vi "Main.vi"() -> ()   [LabVIEW 2021]
uses:
  Type defs/timer Indicator.ctl
  Type defs/Boolean References.ctl
  Type defs/numeric references.ctl
  Type defs/States.ctl
  Type defs/Game Config.ctl
  Type defs/Logs Array.ctl
  <vilib>/Utility/file.llb/Write Delimited Spreadsheet (string).vi
panel:
  in  "increment":bool
  out "Time":string
  in  "Game Config":T1={"Foul Limits"=5.0, "Timeouts Allowed"=5.0, "Game time"=5.0} {"Game time" format="%#_g Min"}
  out "Game Status":enum16{"Paused", "Resumed"}(ring)
  out "Current State":T2
  out "File Status":errorcluster
  out "No. of events Logged":i32
  out "Logging path chosen":path
  out "Logs":string[](array[string])
  in  "Log file path":path
  out "Scores History":dbl[][](graph)
  out "Numeric References":T3
  out "Boolean Refernces":T4
  out "Quarter":dbl
  out "no_timeouts_B":bool
  out "no_timeouts_A":bool
  out "Timeouts_B":dbl
  out "Timeouts_A":dbl
  out "Fouls_Limit B":bool
  out "Fouls_Limit A":bool
  out "Fouls_B":dbl
  out "Fouls_A":dbl
  out "quarter_score_B":dbl[](array[numeric])
  out "quarter_score_A":dbl[](array[numeric])
  out "Score_B":dbl
  out "Score_A":dbl
  in  "Save Logs":bool
  in  "Reset":bool
  in  "Advance Quarter":bool
  in  "Start/Pause":bool
  in  "B_timeout":bool
  in  "B_Foul":bool
  in  "B_3pt":bool
  in  "B_2pt":bool
  in  "B_1pt":bool
  in  "A_timeout":bool
  in  "A_Foul":bool
  in  "A_3pt":bool
  in  "A_2pt":bool
  in  "A_1pt":bool
  out "Timer":T5
  in  "Stop":bool
  # "Game Status"
  # "TEAM B"
  # "TEAM A"
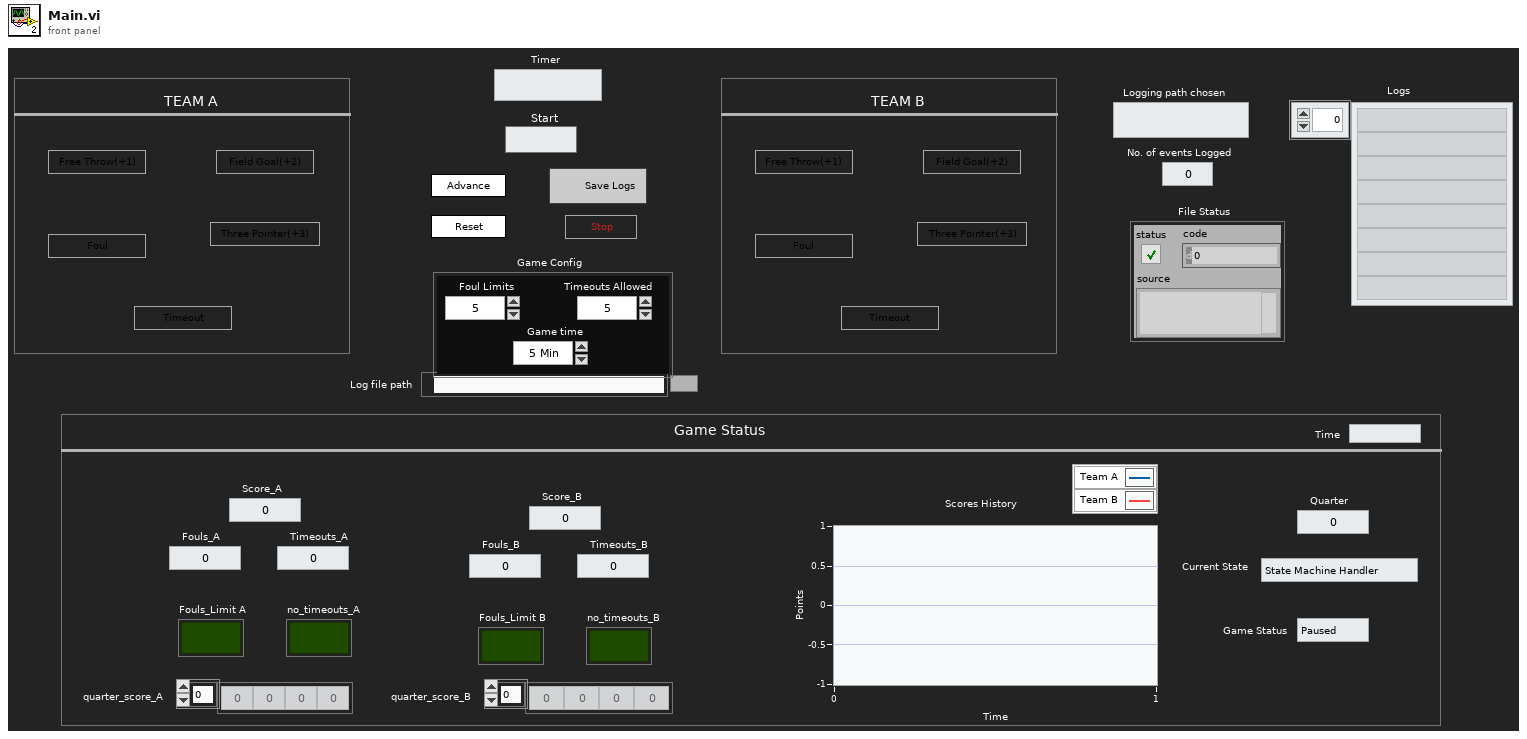
[diagram p1: front panel]
types:
  T1 = typedef "Game Config.ctl" = cluster{"Foul Limits":dbl, "Timeouts Allowed":dbl, "Game time":dbl}
  T2 = typedef "States.ctl" = enum16{"State Machine Handler", "A_1pt", "B_1pt", "A_2pt", "B_2pt", "A_3pt", "B_3pt", "A_Foul", "B_Foul", "A_timeout", "B_timeout", "Next Quarter", "Save Logs", "Reset", "Start/Pause", "Stop"}
  T3 = typedef "numeric references.ctl" = refnum<vi>[]
  T4 = typedef "Boolean References.ctl" = refnum<vi>[]
  T5 = typedef "timer Indicator.ctl" = string
  T6 = typedef "Logs Array.ctl" = string[]
  T7 = enum8{"Enabled", "Disabled", "Disabled and Grayed Out"}
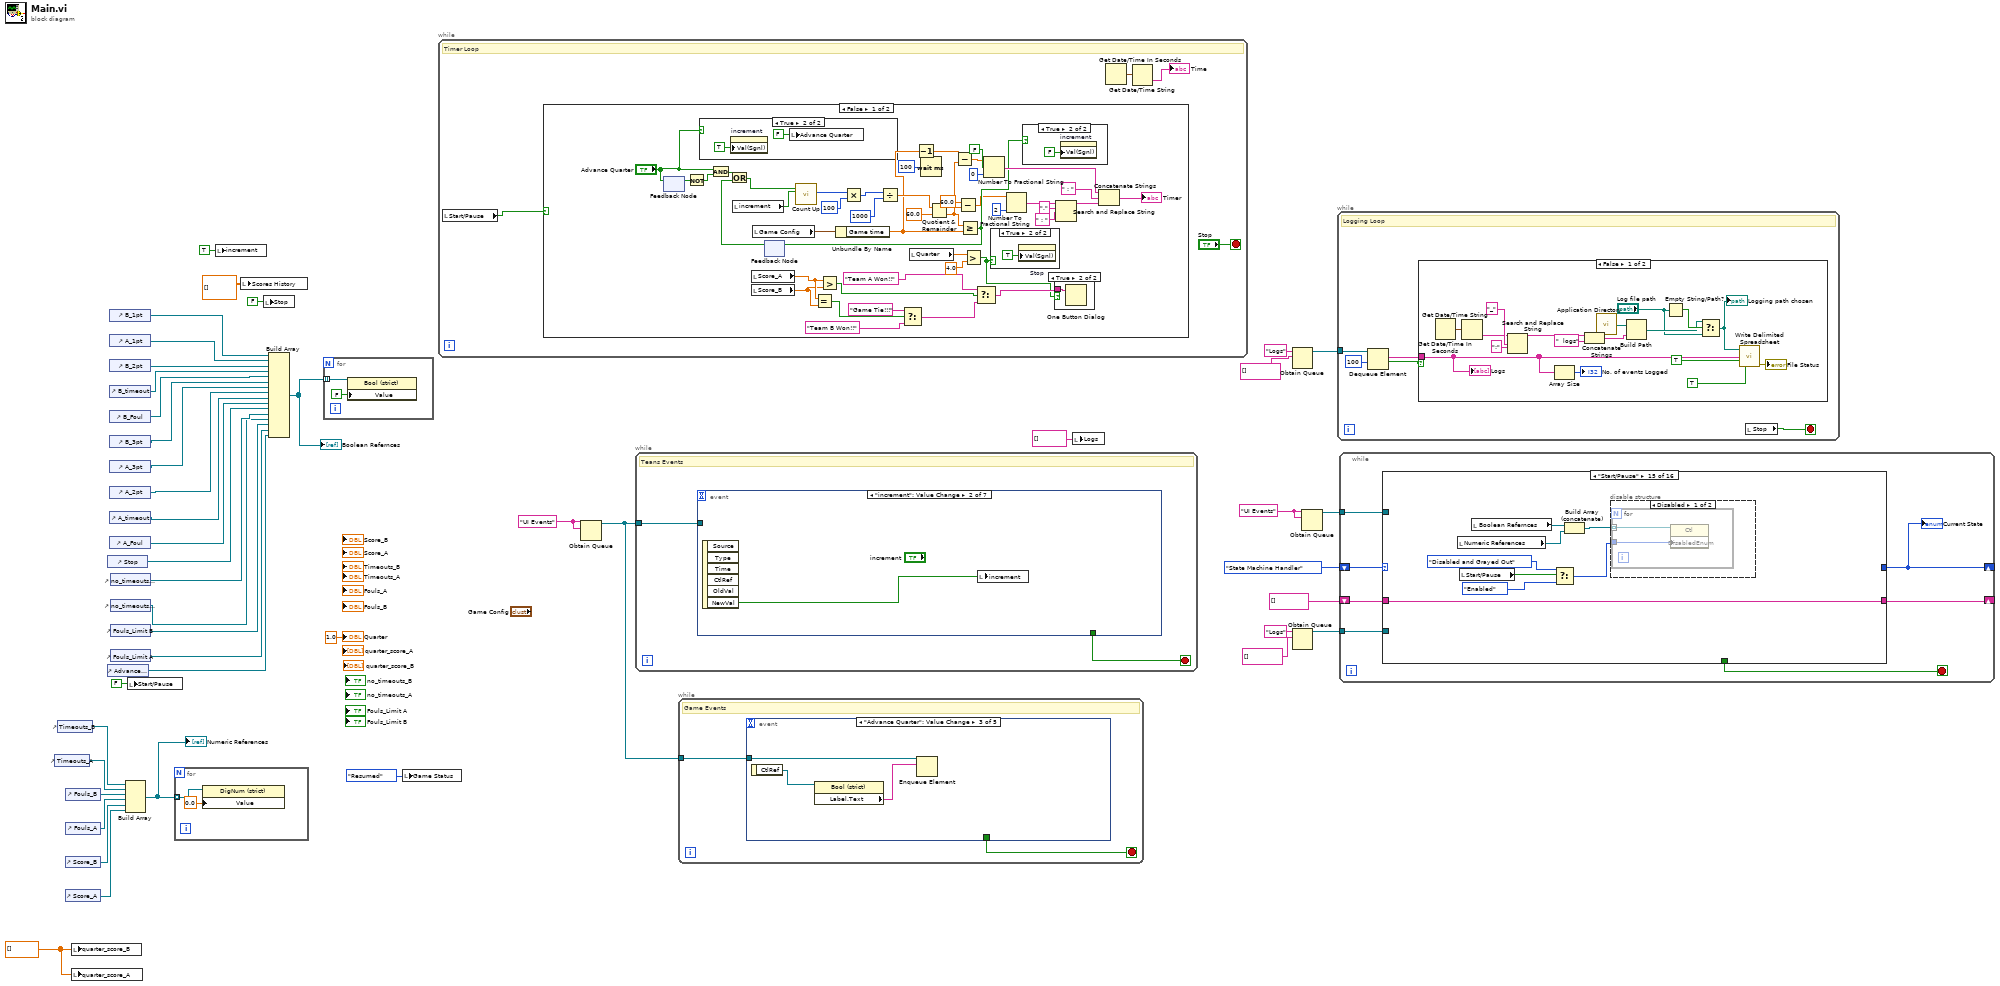
[diagram p0: block diagram]
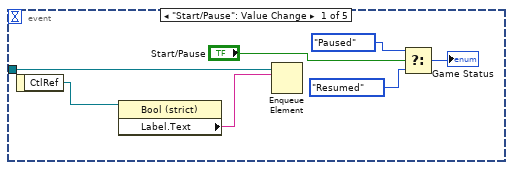
[diagram p2: hidden frame]
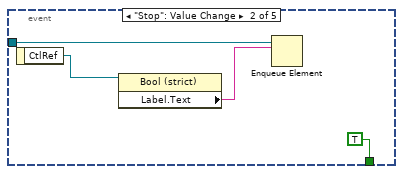
[diagram p3: hidden frame]
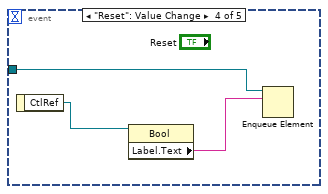
[diagram p4: hidden frame]
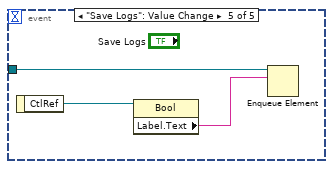
[diagram p5: hidden frame]
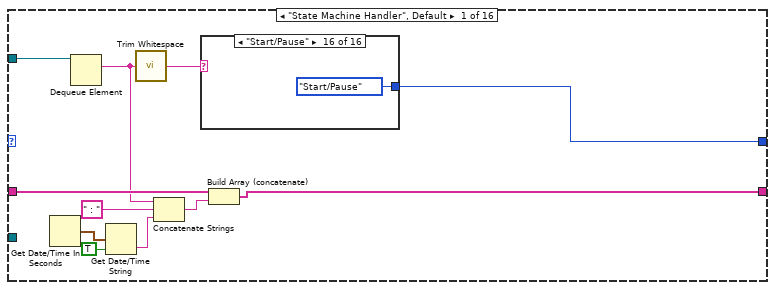
[diagram p6: hidden frame]
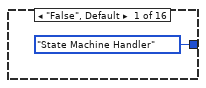
[diagram p7: hidden frame]
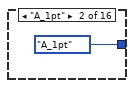
[diagram p8: hidden frame]
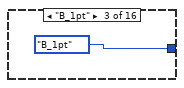
[diagram p9: hidden frame]
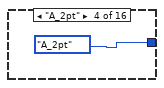
[diagram p10: hidden frame]
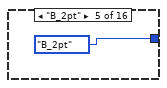
[diagram p11: hidden frame]
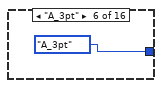
[diagram p12: hidden frame]
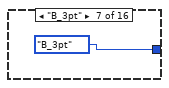
[diagram p13: hidden frame]
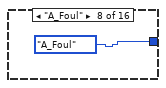
[diagram p14: hidden frame]
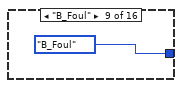
[diagram p15: hidden frame]
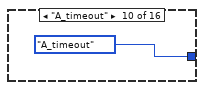
[diagram p16: hidden frame]
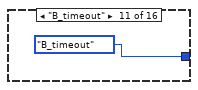
[diagram p17: hidden frame]
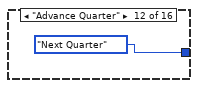
[diagram p18: hidden frame]
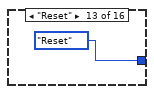
[diagram p19: hidden frame]
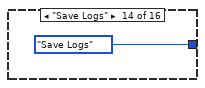
[diagram p20: hidden frame]
diagram:
  w17 = dbl[] [] ("quarter_score_B")
  w32 = "UI Events" ("Label.Text")
  w33 = "UI Events" ("Label.Text")
  n1 = control-ref of="Timeouts_A"() -> (w23:refnum<vi>)
  n2 = control-ref of="Timeouts_B"() -> (w24:refnum<vi>)
  n3 = control-ref of="Fouls_B"() -> (w22:refnum<vi>)
  n4 = control-ref of="Fouls_A"() -> (w21:refnum<vi>)
  n5 = control-ref of="Score_B"() -> (w20:refnum<vi>)
  n6 = control-ref of="Score_A"() -> (w19:refnum<vi>)
  n7 = local write "quarter_score_B"(w17) -> ()
  n8 = local write "quarter_score_A"(w17) -> ()
  n9 = control-ref of="Stop"() -> (w29:refnum<vi>)
  n10 = control-ref of="Advance Quarter"() -> (w3:refnum<vi>)
  n11 = control-ref of="B_1pt"() -> (w44:refnum<vi>)
  n12 = control-ref of="A_1pt"() -> (w43:refnum<vi>)
  n13 = control-ref of="B_2pt"() -> (w42:refnum<vi>)
  n14 = control-ref of="B_timeout"() -> (w41:refnum<vi>)
  n15 = control-ref of="B_Foul"() -> (w40:refnum<vi>)
  n16 = control-ref of="B_3pt"() -> (w39:refnum<vi>)
  n17 = control-ref of="A_3pt"() -> (w38:refnum<vi>)
  n18 = control-ref of="A_2pt"() -> (w37:refnum<vi>)
  n19 = control-ref of="A_timeout"() -> (w36:refnum<vi>)
  n20 = control-ref of="A_Foul"() -> (w35:refnum<vi>)
  n21 = control-ref of="no_timeouts_B"() -> (w28:refnum<vi>)
  n22 = control-ref of="no_timeouts_A"() -> (w27:refnum<vi>)
  n23 = control-ref of="Fouls_Limit B"() -> (w26:refnum<vi>)
  n24 = control-ref of="Fouls_Limit A"() -> (w25:refnum<vi>)
  n25 = Build Array(w24, w23, w22, w21, w20, w19) -> (w18:refnum<vi>[])
  "Numeric References" <- w18
  n26 = local write "Start/Pause"(FALSE ("Start/Pause")) -> ()
  n27 = for {
    tunnel: w18 -> [w46] mode=indexing
    n28 = property class="DigNum (strict)"(reference=w46, "Value"=0.0) -> ()  [unwired: 1 in, 2 out]
  }
  n29 = local write "increment"(TRUE ("increment")) -> ()
  n30 = local write "Scores History"(dbl[][] [] ("Scores History")) -> ()
  n31 = local write "Stop"(FALSE ("Stop")) -> ()
  n32 = Build Array(w44, w43, w42, w41, w40, w39, w38, w37, w36, w35, w29, w28, w27, w26, w25, w3) -> (w34:refnum<vi>[])
  "Boolean Refernces" <- w34
  n33 = for {
    tunnel: w34 -> [w48] mode=indexing
    n34 = property class="Bool (strict)"(reference=w48, "Value"=FALSE) -> ()  [unwired: 1 in, 2 out]
  }
  n35 = local write "Game Status"(enum16{"Paused", "Resumed"}."Resumed" ("Game Status")) -> ()
  n36 = while {
    stop <- "Stop" stop-if-true
    # "Timer Loop"
    n37 = local read "Start/Pause"() -> (w49:bool)
    n38 = case shown="False" w49 {
      frame False {
        n39 = feedback #1() -> (w65:bool)  [unwired: 1 in]
        n40 = feedback-in #1("Advance Quarter") -> ()
        n41 = Not(x=w65) -> (.not. x?=w64:bool)
        n42 = case shown="True" "Advance Quarter" {
          frame False {
          }
          frame True {
            n43 = property on="increment" class="Bool (strict)"("Val(Sgnl)"=TRUE ("Value (Signaling)")) -> ()  [unwired: 2 in, 2 out]
            n44 = local write "Advance Quarter"(FALSE ("Advance Quarter")) -> ()
          }
        }
        n45 = And(x="Advance Quarter", y=w64) -> (x .and. y?=w66:bool)
        n46 = local read "increment"() -> (w60:bool)
        n47 = local read "Score_A"() -> (w80:dbl)
        n48 = local read "Score_B"() -> (w79:dbl)
        n49 = local read "Game Config"() -> (w68:T1)
        n50 = feedback #2() -> (w62:bool)  [unwired: 1 in]
        n51 = Or(x=w66, y=w62) -> (x .or. y?=w67:bool)
        n52 = call "Count Up.vi"("Reset"=w67, "Increment"=w60) -> ("Count"=w74:i32)  [unwired: 9 in]
        n53 = Equal?(x=w80, y=w79) -> (x = y?=w78:bool)
        n54 = Greater?(x=w80, y=w79) -> (0:w81:bool)
        n55 = Unbundle By Name(w68) -> ("Game time"=w59:dbl)
        n56 = Multiply(x=w74, y=100) -> (x*y=w73:i32)
        n57 = Divide(x=w73, y=u32 1000) -> (x/y=w90:dbl)
        n58 = Select(t="Game Tie!!!", s=w78, f="Team B Won!!" ("replace string (\"\")")) -> (s? t:f=w75:string)
        n59 = local read "Quarter"() -> (w71:dbl)
        n60 = Decrement(x=w59) -> (x-1=w53:dbl)
        n61 = Wait (ms)(milliseconds to wait=u32 100) -> ()  [unwired: 1 out]
        n62 = Quotient & Remainder(x=w90, y=60.0) -> (x-y*floor(x/y)=w56:dbl, floor(x/y)=w58:dbl)
        n63 = Subtract(x=w53, y=w58) -> (x-y=w57:dbl)
        n64 = Subtract(x=60.0, y=w56) -> (x-y=w54:dbl)
        n65 = Greater Or Equal?(x=w58, y=w59) -> (x >= y?=w61:bool)
        n66 = feedback-in #2(w61) -> ()
        n67 = Greater?(x=w71, y=4.0) -> (0:w69:bool)
        n68 = Select(t="Team A Won!!" ("replace string (\"\")"), s=w81, f=w75) -> (s? t:f=w82:string)
        n69 = Number To Fractional String(use system decimal point (T)=FALSE, number=w57, precision (6)=i16 0) -> (F-format string=w85:string)  [unwired: 1 in]
        n70 = case shown="True" w69 {
          frame False {
          }
          frame True {
            n71 = property on="Stop" class="Bool (strict)"("Val(Sgnl)"=TRUE ("Value (Signaling)")) -> ()  [unwired: 2 in, 2 out]
          }
        }
        n72 = Number To Fractional String(number=w54, precision (6)=i16 2) -> (F-format string=w94:string)  [unwired: 2 in]
        n73 = case shown="True" w61 {
          frame False {
          }
          frame True {
            n74 = property on="increment" class="Bool (strict)"("Val(Sgnl)"=FALSE ("Value (Signaling)")) -> ()  [unwired: 2 in, 2 out]
          }
        }
        n75 = case shown="True" w69 {
          tunnel: w82 -> [_ w101]
          frame False {
          }
          frame True {
            n76 = One Button Dialog(message=w101) -> ()  [unwired: 1 in, 1 out]
          }
        }
        n77 = Search and Replace String(input string=w94, search string=".", replace string=" : " ("replace string (\"\")")) -> (result string=w91:string)  [unwired: 5 in, 3 out]
        n78 = Concatenate Strings(w85, " : " ("replace string (\"\")"), w91) -> (→"Timer":string)
      }
      frame True {
      }
    }
    n79 = Get Date/Time In Seconds() -> (seconds since 1Jan1904=w51:timestamp)
    n80 = Get Date/Time String(seconds (now)=w51) -> (time string=→"Time":string)  [unwired: 2 in, 1 out]
  }
  n81 = Obtain Queue(name (unnamed)=w33, element data type=w33) -> (queue out=w10:refnum<queue>)  [unwired: 3 in, 2 out]
  n82 = while {
    tunnel: w10 -> [w104]
    stop <- w103 stop-if-true
    # "Teans Events"
    n83 = event shown="[1] \"increment\": Value Change" {
      selector: _ -> [_ _ _ _ _ _ _]
      dyn-events: _ -> [_ _ _ _ _ _ _]
      timeout: _ -> [_ _ _ _ _ _ _]
      tunnel: w104 -> [w107 _ w113 w115 w118 w122 w125]
      tunnel: [w105 _ _ _ _ _ _] -> w103
      event "Stop": Value Change {
        n84 = event-data() -> ("CtlRef"=w106:refnum<vi>)  [unwired: 1 in, 2 out]
        n85 = disable-structure shown="Enabled" {
          disable-tunnel: w107 -> [w109 _]
          disable-tunnel: w106 -> [w108 _]
          frame Enabled {
            n86 = property class="Bool (strict)"(reference=w108) -> ("Label.Text"=w110:string)  [unwired: 1 in, 2 out]
            n87 = Enqueue Element(queue=w109, element=w110) -> ()  [unwired: 2 in, 3 out]
          }
          frame Disabled {
          }
        }
        n88 = local read "Stop"() -> (w105:bool)
      }
      event "increment": Value Change {
        n89 = event-data() -> ("NewVal"=w111:bool)  [unwired: 1 in, 5 out]
        n90 = local write "increment"(w111) -> ()
      }
      event "A_1pt", "B_1pt": Value Change {
        n91 = event-data() -> ("CtlRef"=w114:refnum<vi>)  [unwired: 1 in]
        n92 = property class="Bool (strict)"(reference=w114) -> ("Label.Text"=w112:string)  [unwired: 1 in, 2 out]
        n93 = Enqueue Element(queue=w113, element=w112) -> ()  [unwired: 2 in, 3 out]
      }
      event "A_2pt", "B_2pt": Value Change {
        n94 = event-data() -> ("CtlRef"=w116:refnum<vi>)  [unwired: 1 in, 2 out]
        n95 = property class="Bool (strict)"(reference=w116) -> ("Label.Text"=w117:string)  [unwired: 1 in, 2 out]
        n96 = Enqueue Element(queue=w115, element=w117) -> ()  [unwired: 2 in, 3 out]
      }
      event "A_3pt", "B_3pt": Value Change {
        n97 = event-data() -> ("CtlRef"=w119:refnum<vi>)  [unwired: 1 in, 2 out]
        n98 = property class="Bool (strict)"(reference=w119) -> ("Label.Text"=w120:string)  [unwired: 1 in, 2 out]
        n99 = Enqueue Element(queue=w118, element=w120) -> ()  [unwired: 2 in, 3 out]
      }
      event "A_Foul", "B_Foul": Value Change {
        n100 = event-data() -> ("CtlRef"=w121:refnum<vi>)  [unwired: 1 in, 2 out]
        n101 = property class="Bool (strict)"(reference=w121) -> ("Label.Text"=w123:string)  [unwired: 1 in, 2 out]
        n102 = Enqueue Element(queue=w122, element=w123) -> ()  [unwired: 2 in, 3 out]
      }
      event "A_timeout", "B_timeout": Value Change {
        n103 = event-data() -> ("CtlRef"=w124:refnum<vi>)  [unwired: 1 in, 2 out]
        n104 = property class="Bool (strict)"(reference=w124) -> ("Label.Text"=w126:string)  [unwired: 1 in, 2 out]
        n105 = Enqueue Element(queue=w125, element=w126) -> ()  [unwired: 2 in, 3 out]
      }
    }
  }
  n106 = while {
    tunnel: w10 -> [w128]
    stop <- w127 stop-if-true
    # "Game Events"
    n107 = event shown="[2] \"Advance Quarter\": Value Change" {
      selector: _ -> [_ _ _ _ _]
      dyn-events: _ -> [_ _ _ _ _]
      timeout: _ -> [_ _ _ _ _]
      tunnel: w128 -> [w133 w137 w140 w144 w147]
      tunnel: [_ TRUE _ _ _] -> w127
      event "Start/Pause": Value Change {
        n108 = event-data() -> ("CtlRef"=w134:refnum<vi>)  [unwired: 1 in]
        n109 = property class="Bool (strict)"(reference=w134) -> ("Label.Text"=w135:string)  [unwired: 1 in, 2 out]
        n110 = Enqueue Element(queue=w133, element=w135) -> ()  [unwired: 2 in, 3 out]
        n111 = Select(t=enum16{"Paused", "Resumed"}."Paused", s="Start/Pause", f=enum16{"Paused", "Resumed"}."Resumed") -> (s? t:f=→"Game Status":enum16{"Paused", "Resumed"})
      }
      event "Stop": Value Change {
        n112 = event-data() -> ("CtlRef"=w138:refnum<vi>)  [unwired: 1 in]
        n113 = property class="Bool (strict)"(reference=w138) -> ("Label.Text"=w139:string)  [unwired: 1 in, 2 out]
        n114 = Enqueue Element(queue=w137, element=w139) -> ()  [unwired: 2 in, 3 out]
      }
      event "Advance Quarter": Value Change {
        n115 = event-data() -> ("CtlRef"=w141:refnum<vi>)  [unwired: 1 in]
        n116 = property class="Bool (strict)"(reference=w141) -> ("Label.Text"=w142:string)  [unwired: 1 in, 2 out]
        n117 = Enqueue Element(queue=w140, element=w142) -> ()  [unwired: 2 in, 3 out]
      }
      event "Reset": Value Change {
        n118 = event-data() -> ("CtlRef"=w143:refnum<vi>)  [unwired: 1 in]
        n119 = property class="Bool"(reference=w143) -> ("Label.Text"=w145:string)  [unwired: 1 in, 2 out]
        n120 = Enqueue Element(queue=w144, element=w145) -> ()  [unwired: 2 in, 3 out]
      }
      event "Save Logs": Value Change {
        n121 = event-data() -> ("CtlRef"=w146:refnum<vi>)  [unwired: 1 in]
        n122 = property class="Bool"(reference=w146) -> ("Label.Text"=w148:string)  [unwired: 1 in, 2 out]
        n123 = Enqueue Element(queue=w147, element=w148) -> ()  [unwired: 2 in, 3 out]
      }
    }
  }
  n124 = local write "Logs"(string[] [] ("Logs")) -> ()
  n125 = Obtain Queue(name (unnamed)="Logs", element data type=T6 []) -> (queue out=w11:refnum<queue>)  [unwired: 3 in, 2 out]
  n126 = Obtain Queue(name (unnamed)="Logs", element data type=T6 []) -> (queue out=w13:refnum<queue>)  [unwired: 3 in, 2 out]
  n127 = Obtain Queue(name (unnamed)=w32, element data type=w32) -> (queue out=w31:refnum<queue>)  [unwired: 3 in, 2 out]
  n128 = while {
    tunnel: w11 -> [w152]
    stop <- w153 stop-if-true
    # "Logging Loop"
    n129 = Dequeue Element(queue=w152, timeout in ms (-1)=100) -> (element=w150:T6, timed out?=w151:bool)  [unwired: 1 in, 2 out]
    n130 = case shown="False" w151 {
      tunnel: w150 -> [w156 _]
      frame False {
        n131 = Get Date/Time In Seconds() -> (seconds since 1Jan1904=w164:timestamp)
        n132 = Get Date/Time String(seconds (now)=w164) -> (time string=w165:string)  [unwired: 2 in, 1 out]
        n133 = Search and Replace String(input string=w165, search string=":", replace string="_" ("replace string (\"\")")) -> (result string=w168:string)  [unwired: 5 in, 3 out]
        n134 = Array Size(array=w156) -> (size(s)=→"No. of events Logged":i32)
        n135 = Concatenate Strings(w168, "  logs" ("string")) -> (w169:string)
        n136 = call <vilib>:"Application Directory.vi"() -> ("Application Directory"=w163:path)
        n137 = Build Path(base path=w163, name or relative path=w169) -> (appended path=w159:path)
        n138 = Empty String/Path?(string/path="Log file path") -> (empty?=w160:bool)
        n139 = Select(t=w159, s=w160, f="Log file path") -> (s? t:f=w157:path)
        "Logging path chosen" <- w157
        n140 = call-poly <vilib>:"Write Delimited Spreadsheet.vi"("file path (dialog if empty)"=w157, "1D data"=w156, "append to file? (new file:F)"=TRUE, "transpose? (no:F)"=TRUE) -> ("error out"=→"File Status":errorcluster)  [unwired: 10 in, 1 out]
        "Logs" <- w156
      }
      frame True {
      }
    }
    n141 = local read "Stop"() -> (w153:bool)
  }
  n142 = while {
    tunnel: w31 -> [w176]
    shift-right: [w175] -> _
    shift-left: States."State Machine Handler" -> [w177]
    shift-right: [w173] -> _
    shift-left: string[] [] -> [w172]
    tunnel: w13 -> [w171]
    stop <- w174 stop-if-true
    n143 = case shown="\"Start/Pause\"" w177 {
      tunnel: w176 -> [w188 _ _ _ _ _ _ _ _ _ _ _ _ _ _ _]
      tunnel: [w187 _ _ _ _ _ _ _ _ _ _ _ _ _ _ States."State Machine Handler"] -> w175
      tunnel: [_ _ _ _ _ _ _ _ _ _ _ _ _ _ _ TRUE ("Stop")] -> w174
      tunnel: [w181 w206 w211 w216 w221 w226 w231 w242 w249 w255 w264 w286 w293 _ w305 w317] -> w173
      tunnel: w172 -> [w185 w206 w211 w216 w221 w226 w231 w242 w249 w255 w264 w286 w293 _ w305 w317]
      tunnel: w171 -> [_ _ _ _ _ _ _ _ _ _ _ _ w294 _ _ _]
      frame "State Machine Handler", Default {
        n144 = Get Date/Time In Seconds() -> (seconds since 1Jan1904=w183:timestamp)
        n145 = Dequeue Element(queue=w188) -> (element=w184:string)  [unwired: 2 in, 3 out]
        n146 = Get Date/Time String(seconds (now)=w183, want seconds? (F)=TRUE) -> (time string=w179:string)  [unwired: 1 in, 1 out]
        n147 = call <vilib>:"Trim Whitespace.vi"("string"=w184) -> ("trimmed string"=w186:string)  [unwired: 1 in]
        n148 = Concatenate Strings(w184, " : " ("element"), w179) -> (w178:string)
        n149 = case shown="\"Start/Pause\"" w186 {
          tunnel: [States."State Machine Handler" States."A_1pt" States."B_1pt" States."A_2pt" States."B_2pt" States."A_3pt" States."B_3pt" States."A_Foul" States."B_Foul" States."A_timeout" States."B_timeout" States."Next Quarter" States."Reset" States."Save Logs" States."Stop" States."Start/Pause"] -> w187
          frame "False", Default {
          }
          frame "A_1pt" {
          }
          frame "B_1pt" {
          }
          frame "A_2pt" {
          }
          frame "B_2pt" {
          }
          frame "A_3pt" {
          }
          frame "B_3pt" {
          }
          frame "A_Foul" {
          }
          frame "B_Foul" {
          }
          frame "A_timeout" {
          }
          frame "B_timeout" {
          }
          frame "Advance Quarter" {
          }
          frame "Reset" {
          }
          frame "Save Logs" {
          }
          frame "Stop" {
          }
          frame "Start/Pause" {
          }
        }
        n150 = Build Array (concatenate)(w185, w178) -> (w181:string[])
      }
      frame "A_1pt" {
        n151 = local read "Score_A"() -> (w209:dbl)
        n152 = call "Add.vi"("Add value"=1.0, "Score_A"=w209) -> ("Score Out"=w207:dbl)  [unwired: 9 in]
        n153 = local write "A_1pt"(FALSE ("A_1pt")) -> ()
        n154 = local write "Score_A"(w207) -> ()
      }
      frame "B_1pt" {
        n155 = local read "Score_B"() -> (w214:dbl)
        n156 = call "Add.vi"("Add value"=1.0, "Score_A"=w214) -> ("Score Out"=w212:dbl)  [unwired: 9 in]
        n157 = local write "B_1pt"(FALSE ("B_1pt")) -> ()
        n158 = local write "Score_B"(w212) -> ()
      }
      frame "A_2pt" {
        n159 = local read "Score_A"() -> (w219:dbl)
        n160 = local write "A_2pt"(FALSE ("A_2pt")) -> ()
        n161 = call "Add.vi"("Add value"=2.0, "Score_A"=w219) -> ("Score Out"=w217:dbl)  [unwired: 9 in]
        n162 = local write "Score_A"(w217) -> ()
      }
      frame "B_2pt" {
        n163 = local read "Score_B"() -> (w224:dbl)
        n164 = local write "B_2pt"(FALSE ("B_2pt")) -> ()
        n165 = call "Add.vi"("Add value"=2.0, "Score_A"=w224) -> ("Score Out"=w222:dbl)  [unwired: 9 in]
        n166 = local write "Score_B"(w222) -> ()
      }
      frame "A_3pt" {
        n167 = local read "Score_A"() -> (w229:dbl)
        n168 = call "Add.vi"("Add value"=3.0, "Score_A"=w229) -> ("Score Out"=w227:dbl)  [unwired: 9 in]
        n169 = local write "A_3pt"(FALSE ("A_3pt")) -> ()
        n170 = local write "Score_A"(w227) -> ()
      }
      frame "B_3pt" {
        n171 = local read "Score_B"() -> (w234:dbl)
        n172 = call "Add.vi"("Add value"=3.0, "Score_A"=w234) -> ("Score Out"=w232:dbl)  [unwired: 9 in]
        n173 = local write "B_3pt"(FALSE ("B_3pt")) -> ()
        n174 = local write "Score_B"(w232) -> ()
      }
      frame "A_Foul" {
        n175 = local read "Game Config"() -> (w236:T1)
        n176 = Unbundle By Name(w236) -> ("Foul Limits"=w235:dbl)
        n177 = local read "Fouls_A"() -> (w240:dbl)
        n178 = local write "A_Foul"(FALSE ("A_Foul")) -> ()
        n179 = call "Add_foul.vi"("Add value"=1.0, "Score_A"=w240) -> ("Score Out"=w238:dbl)  [unwired: 9 in]
        n180 = Greater?(x=w238, y=w235) -> (0:w237:bool)
        n181 = local write "Fouls_A"(w238) -> ()
        n182 = local write "Fouls_Limit A"(w237) -> ()
      }
      frame "B_Foul" {
        n183 = local read "Game Config"() -> (w244:T1)
        n184 = local write "B_Foul"(FALSE ("B_Foul")) -> ()
        n185 = local read "Fouls_B"() -> (w248:dbl)
        n186 = Unbundle By Name(w244) -> ("Foul Limits"=w243:dbl)
        n187 = call "Add_foul.vi"("Add value"=1.0, "Score_A"=w248) -> ("Score Out"=w245:dbl)  [unwired: 9 in]
        n188 = local write "Fouls_B"(w245) -> ()
        n189 = Greater?(x=w245, y=w243) -> (0:w246:bool)
        n190 = local write "Fouls_Limit B"(w246) -> ()
      }
      frame "A_timeout" {
        n191 = local read "Game Config"() -> (w254:T1)
        n192 = local read "Timeouts_A"() -> (w257:dbl)
        n193 = local write "A_timeout"(FALSE ("A_timeout")) -> ()
        n194 = Unbundle By Name(w254) -> ("Timeouts Allowed"=w251:dbl)
        n195 = call "Add_timeouts.vi"("Add value"=1.0, "Score_A"=w257) -> ("Score Out"=w253:dbl)  [unwired: 9 in]
        n196 = Greater?(x=w253, y=w251) -> (0:w252:bool)
        n197 = case shown="False" w252 {
          tunnel: w253 -> [w259 _]
          frame False {
            n198 = local write "Timeouts_A"(w259) -> ()
          }
          frame True {
          }
        }
        n199 = local write "no_timeouts_A"(w252) -> ()
      }
      frame "B_timeout" {
        n200 = local read "Game Config"() -> (w261:T1)
        n201 = local read "Timeouts_B"() -> (w266:dbl)
        n202 = local write "B_timeout"(FALSE ("B_timeout")) -> ()
        n203 = Unbundle By Name(w261) -> ("Timeouts Allowed"=w260:dbl)
        n204 = call "Add_timeouts.vi"("Add value"=1.0, "Score_A"=w266) -> ("Score Out"=w262:dbl)  [unwired: 9 in]
        n205 = Greater?(x=w262, y=w260) -> (0:w263:bool)
        n206 = case shown="False" w263 {
          tunnel: w262 -> [w268 _]
          frame False {
            n207 = local write "Timeouts_B"(w268) -> ()
          }
          frame True {
          }
        }
        n208 = local write "no_timeouts_B"(w263) -> ()
      }
      frame "Next Quarter" {
        n209 = local read "Quarter"() -> (w288:dbl)
        n210 = local read "quarter_score_A"() -> (w285:dbl[])
        n211 = local read "quarter_score_B"() -> (w284:dbl[])
        n212 = local read "Score_A"() -> (w273:dbl)
        n213 = local read "Score_B"() -> (w274:dbl)
        n214 = call "Add_quarter.vi"("Add value"=1.0, "Score_A"=w288) -> ("Score Out"=w280:dbl)  [unwired: 9 in]
        n215 = Greater?(x=w280, y=4.0) -> (0:w275:bool)
        n216 = Greater?(x=w273, y=w274) -> (0:w278:bool)
        n217 = local write "Quarter"(w280) -> ()
        n218 = case shown="True" w275 {
          frame False {
          }
          frame True {
            n219 = property on="Stop" class="Bool (strict)"("Val(Sgnl)"=TRUE ("Value (Signaling)")) -> ()  [unwired: 2 in, 2 out]
          }
        }
        n220 = Equal?(x=w273, y=w274) -> (x = y?=w272:bool)
        n221 = call "graph make.vi"("Score_B"=w274, "quarter_score_B"=w284, "Score_A"=w273, "quarter_score_A"=w285) -> ("Array 2"=w282:dbl[], "Array"=w281:dbl[][], "Array 3"=w283:dbl[])  [unwired: 5 in]
        "Scores History" <- w281
        n222 = Select(t="Game Tie!!!", s=w272, f="Team B Won!!" ("replace string (\"\")")) -> (s? t:f=w269:string)
        n223 = Select(t="Team A Won!!" ("replace string (\"\")"), s=w278, f=w269) -> (s? t:f=w276:string)
        n224 = case shown="True" w275 {
          tunnel: w276 -> [_ w289]
          frame False {
          }
          frame True {
            n225 = One Button Dialog(message=w289) -> ()  [unwired: 1 in, 1 out]
          }
        }
        n226 = local write "quarter_score_A"(w283) -> ()
        n227 = local write "quarter_score_B"(w282) -> ()
        n228 = flat-sequence {
          tunnel: w281 -> [_]
          frame #0 {
            n229 = local write "Fouls_A"(0.0 ("Score_B")) -> ()
            n230 = local write "Fouls_B"(0.0 ("Score_A")) -> ()
          }
        }
      }
      frame "Save Logs" {
        n231 = Enqueue Element(queue=w294, element=w293) -> ()  [unwired: 2 in, 3 out]
      }
      frame "Reset" {
        w300 = dbl[] [] ("quarter_score_B")
        n232 = local read "Numeric References"() -> (w298:T3)
        n233 = local read "Boolean Refernces"() -> (w299:T4)
        n234 = local write "quarter_score_B"(w300) -> ()
        n235 = local write "quarter_score_A"(w300) -> ()
        n236 = for {
          tunnel: w298 -> [w302] mode=indexing
          n237 = property class="DigNum (strict)"(reference=w302, "Value"=0.0) -> ()  [unwired: 1 in, 2 out]
        }
        n238 = for {
          tunnel: w299 -> [w304] mode=indexing
          n239 = property class="Bool (strict)"(reference=w304, "Value"=FALSE) -> ()  [unwired: 1 in, 2 out]
        }
        n240 = local write "No. of events Logged"(0 ("No. of events Logged")) -> ()
        n241 = local write "Quarter"(1.0 ("Quarter")) -> ()
        n242 = local write "Logs"(string[] [] ("Logs")) -> ()
      }
      frame "Start/Pause" {
        n243 = local read "Numeric References"() -> (w310:T3)
        n244 = local read "Start/Pause"() -> (w309:bool)
        n245 = local read "Boolean Refernces"() -> (w312:T4)
        n246 = Select(t=T7."Disabled and Grayed Out" ("Disabled"), s=w309, f=T7."Enabled") -> (s? t:f=w306:T7)
        n247 = Build Array (concatenate)(w312, w310) -> (w311:refnum<vi>[])
        n248 = disable-structure shown="Disabled" {
          disable-tunnel: w311 -> [w314 _]
          disable-tunnel: w306 -> [w313 _]
          frame Disabled {
            n249 = for {
              tunnel: w314 -> [w316] mode=indexing
              tunnel: w313 -> [w315]
              n250 = property class="Ctl"(reference=w316, "DisabledEnum"=w315) -> ()  [unwired: 1 in, 2 out]
            }
          }
          frame Enabled {
          }
        }
      }
      frame "Stop" {
      }
    }
    "Current State" <- w175
  }
  "Quarter" <- 1.0 ("Quarter")
